vi "MotorSimulator.vi"(5 "Commanded RPM":dbl, 9 "Load (%)":dbl) -> (4 "Measurements":T1)   [LabVIEW 2026]
uses:
  MotorMeasurements.ctl
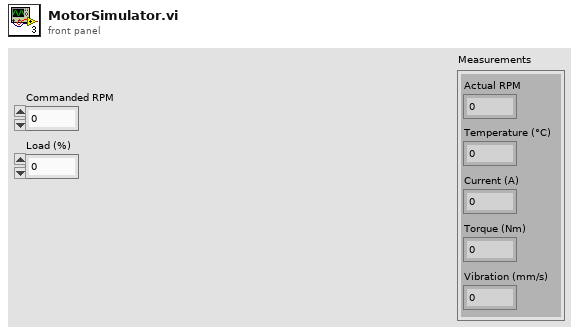
[diagram p1: front panel]
types:
  T1 = typedef "MotorMeasurements.ctl" = cluster{"Temperature (°C)":dbl, "Current (A)":dbl, "Torque (Nm)":dbl, "Vibration (mm/s)":dbl, "Actual RPM":dbl}
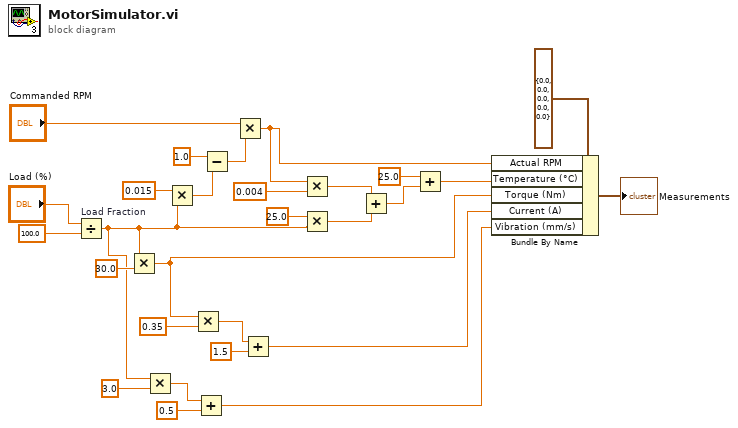
[diagram p0: block diagram]
diagram:
  n1 = Divide "Load Fraction"(x="Load (%)", y=100.0) -> (x/y=w11:dbl)
  n2 = Multiply(x=w11, y=30.0) -> (x*y=w3:dbl)
  n3 = Multiply(x=w11, y=3.0) -> (x*y=w8:dbl)
  n4 = Multiply(x=0.015, y=w11) -> (x*y=w23:dbl)
  n5 = Multiply(x=w3, y=0.35) -> (x*y=w19:dbl)
  n6 = Add(x=w8, y=0.5) -> (x+y=w1:dbl)
  n7 = Subtract(x=1.0, y=w23) -> (x-y=w22:dbl)
  n8 = Multiply(x="Commanded RPM", y=w22) -> (x*y=w7:dbl)
  n9 = Add(x=w19, y=1.5) -> (x+y=w2:dbl)
  n10 = Multiply(x=w7, y=0.004) -> (x*y=w15:dbl)
  n11 = Multiply(x=25.0, y=w11) -> (x*y=w14:dbl)
  n12 = Add(x=w15, y=w14) -> (x+y=w13:dbl)
  n13 = Add(x=25.0, y=w13) -> (x+y=w4:dbl)
  n14 = Bundle By Name(cluster=T1 {"Temperature (°C)"=0.0, "Current (A)"=0.0, "Torque (Nm)"=0.0, "Vibration (mm/s)"=0.0, "Actual RPM"=0.0} ("Measurements"), "Actual RPM"=w7, "Temperature (°C)"=w4, "Torque (Nm)"=w3, "Current (A)"=w2, "Vibration (mm/s)"=w1) -> (→"Measurements":T1)
